vi "2.vi"() -> ()   [LabVIEW 2013]
panel:
  out "Sort Array":dbl[](array[numeric])
  out "Array":dbl[](array[numeric])
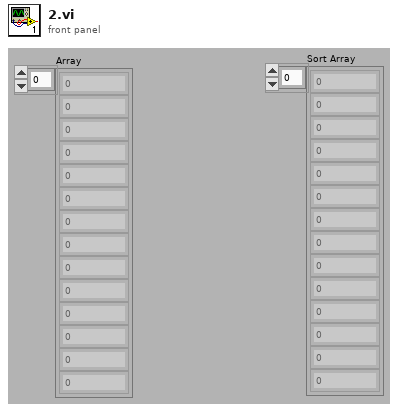
[diagram p1: front panel]
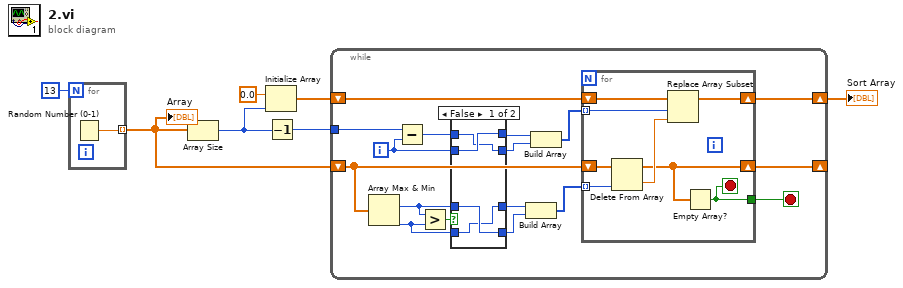
[diagram p0: block diagram]
diagram:
  n1 = for {
    N: 13 -> [_]
    tunnel: [w8] -> w4 mode=indexing
    n2 = Random Number (0-1)() -> (number: 0 to 1=w8:dbl)
  }
  "Array" <- w4
  n3 = Array Size(array=w4) -> (size(s)=w3:i32)
  n4 = Initialize Array(0.0 ("element"), w3) -> (w5:dbl[])
  n5 = Decrement(x=w3) -> (x-1=w2:i32)
  n6 = while {
    shift-right: [w11] -> _
    shift-left: w4 -> [w25]
    shift-right: [w23] -> w1
    shift-left: w5 -> [w24]
    tunnel: w2 -> [w17]
    i -> [w15]
    stop <- w10 stop-if-true
    n7 = Array Max & Min(array=w25) -> (max index (indices)=w21:i32, min index (indices)=w20:i32)  [unwired: 2 out]
    n8 = Subtract(x=w17, y=w15) -> (x-y=w16:i32)
    n9 = Greater?(x=w21, y=w20) -> (0:w22:bool)
    n10 = case shown="False" w22 {
      tunnel: w21 -> [w37 w41]
      tunnel: [w36 w41] -> w19
      tunnel: w20 -> [w36 w40]
      tunnel: [w37 w40] -> w18
      tunnel: w16 -> [w34 w39]
      tunnel: w15 -> [w35 w38]
      tunnel: [w35 w39] -> w13
      tunnel: [w34 w38] -> w14
      frame False {
      }
      frame True {
      }
    }
    n11 = Build Array(w19, w18) -> (w9:i32[])
    n12 = Build Array(w13, w14) -> (w12:i32[])
    n13 = for {
      tunnel: w12 -> [w29] mode=indexing
      shift-right: [w31] -> w23
      shift-left: w24 -> [w32]
      tunnel: w9 -> [w28] mode=indexing
      shift-right: [w27] -> w11
      shift-left: w25 -> [w33]
      tunnel: [w26] -> w10
      stop <- w26 stop-if-true
      n14 = Delete From Array(array=w33, index=w28) -> (deleted portion=w30:dbl, array with subset deleted=w27:dbl[])  [unwired: 1 in]
      n15 = Replace Array Subset(array=w32, new element=w30, index=w29) -> (w31:dbl[])
      n16 = Empty Array?(array=w27) -> (empty?=w26:bool)
    }
  }
  "Sort Array" <- w1
